vi "API - Stream - Stop Data Streaming from Device.vi"(8 "error in":errorcluster, 11 "DAQiFi Device Properties In":T1) -> (0 "error out":errorcluster, 3 "DAQiFi Device Properties Out":T1)   [LabVIEW 2021]
doc: "Send a command to the DAQ device which stops the data streaming."
uses:
  TypeDefs/TypeDef - Cluster of DAQiFi Device Properties.ctl
  TypeDefs/Enum - Connection Type.ctl
  TCP - Asynchronous Write.vi
  USB - Asynchronous Write.vi
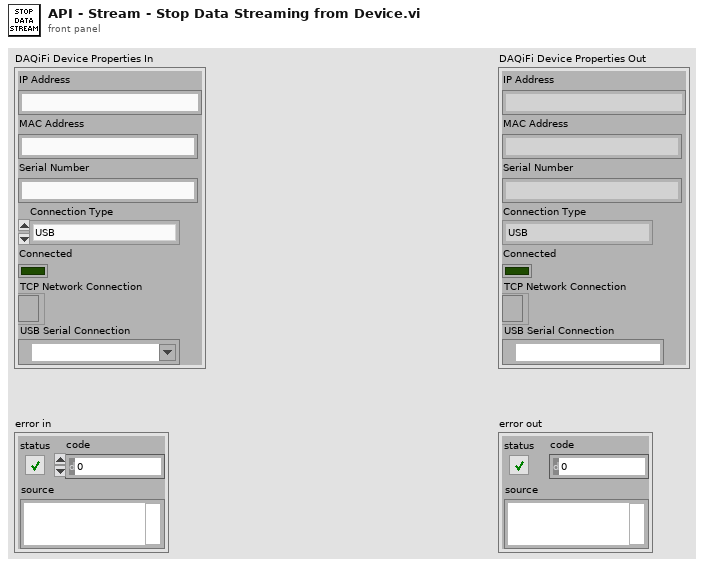
[diagram p1: front panel]
types:
  T1 = typedef "TypeDef - Cluster of DAQiFi Device Properties.ctl" = cluster{"IP Address":string, "MAC Address":string, "Serial Number":string, "Connection Type":T2, "Connected":bool, "TCP Network Connection":refnum<k5>, "USB Serial Connection":refnum<visa-resource-name>}
  T2 = typedef "Enum - Connection Type.ctl" = enum16{"USB", "TCP"}
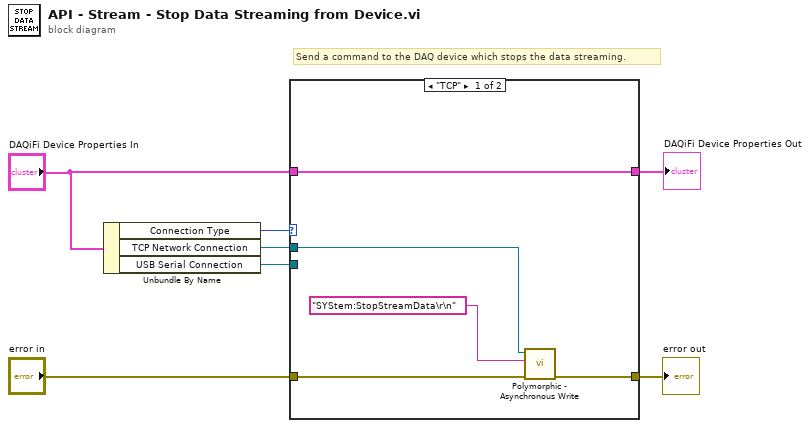
[diagram p0: block diagram]
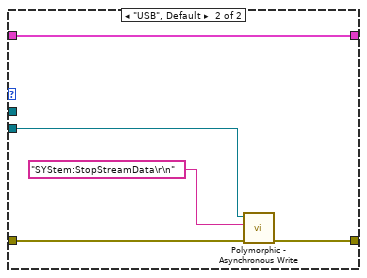
[diagram p2: hidden frame]
diagram:
  # "Send a command to the DAQ device which stops the data streaming."
  n1 = Unbundle By Name("DAQiFi Device Properties In") -> ("Connection Type"=w5:T2, "TCP Network Connection"=w4:refnum<k5>, "USB Serial Connection"=w3:refnum<visa-resource-name>)
  n2 = case shown="\"TCP\"" w5 {
    tunnel: "error in" -> [w12 w17]
    tunnel: [w11 w16] -> w6
    tunnel: w4 -> [w9 _]
    tunnel: w3 -> [_ w14]
    tunnel: [w8 w13] -> w1
    tunnel: "DAQiFi Device Properties In" -> [w8 w13]
    frame "TCP" {
      n3 = call-poly "Polymorphic - Asynchronous Write.vi"("error in"=w12, "Message to Send"="SYStem:StopStreamData\r\n", "TCP Network Connection in"=w9) -> ("error out"=w11:errorcluster)  [unwired: 7 in, 1 out]
    }
    frame "USB", Default {
      n4 = call-poly "Polymorphic - Asynchronous Write.vi"("error in"=w17, "Message to Send"="SYStem:StopStreamData\r\n", "VISA resource name in"=w14) -> ("error out"=w16:errorcluster)  [unwired: 7 in, 1 out]
    }
  }
  "error out" <- w6
  "DAQiFi Device Properties Out" <- w1
